vi "제목없음 2.vi"() -> ()   [LabVIEW 2017]
uses:
  <vilib>/DAQmx/read.llb/DAQmx Read (Analog Wfm 1Chan NSamp).vi
  <vilib>/DAQmx/create/channels.llb/DAQmx Create Channel (AI-Voltage-Basic).vi
  <vilib>/DAQmx/configure/timing.llb/DAQmx Timing (Sample Clock).vi
  <vilib>/DAQmx/miscellaneous.llb/DAQmx Fill In Error Info.vi
panel:
  out "RX.CH2":waveform(dbl)(graph)
  in  "sampling rate":dbl=192000.0 caption="Sampling Frequency" format="%0.2f"
  in  "RX Time(sec)":dbl=0.2
  in  "Number of Sample":i32=19200
  in  "수신 채널 설정":tag="Dev3/ai0:1"
  in  "수신 디바이스 이름":tag="Dev3"
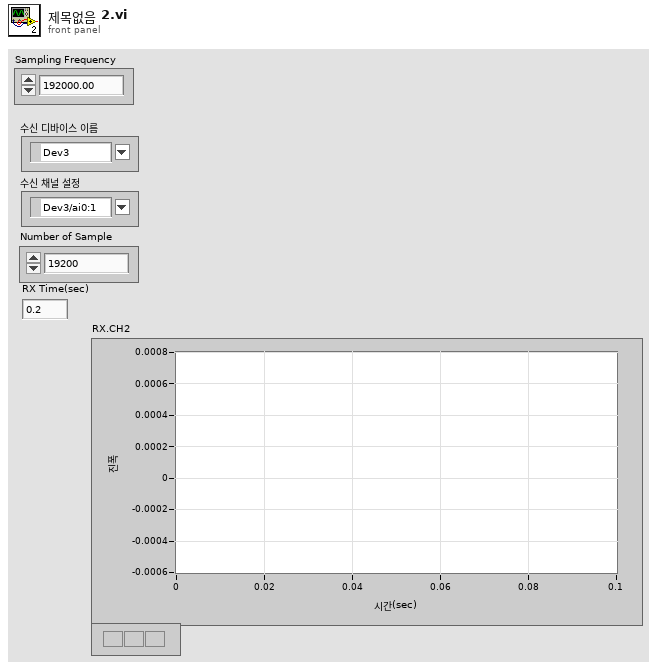
[diagram p1: front panel]
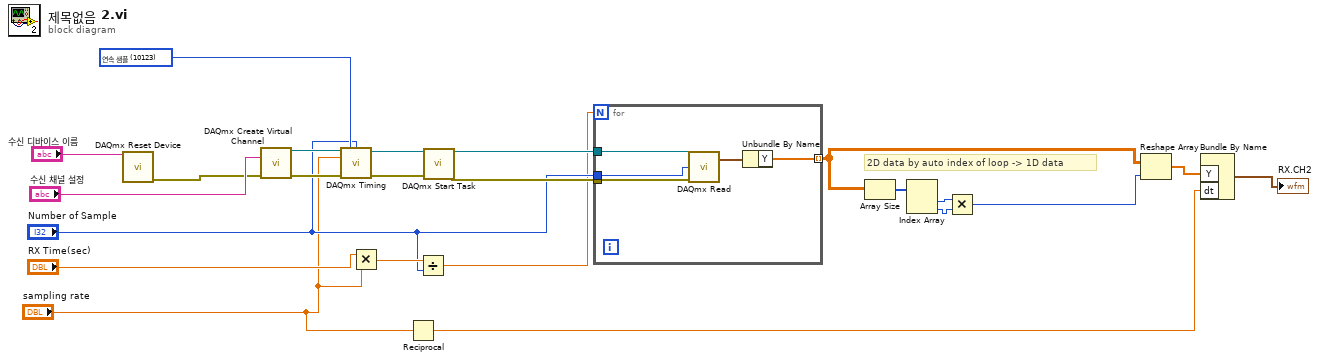
[diagram p0: block diagram]
diagram:
  w14 = 10123 items=["유한 샘플"=10178, "연속 샘플"=10123, "하드웨어 타이밍에 의한 단일 포인트"=12522] ("sample mode")
  # "2D data by auto index of loop -> 1D data"
  n1 = call <vilib>:"DAQmx Reset Device.vi"("device in"="수신 디바이스 이름") -> ("error out"=w20:errorcluster)  [unwired: 1 in, 13 out]
  n2 = call-poly <vilib>:"DAQmx Create Virtual Channel.vi"("physical channels"="수신 채널 설정", "error in"=w20) -> ("task out"=w22:refnum<k21>, "error out"=w19:errorcluster)  [unwired: 7 in, 5 out]
  n3 = call-poly <vilib>:"DAQmx Timing.vi"("task/channels in"=w22, "sample mode"=w14, "samples per channel"="Number of Sample", "rate"="sampling rate", "error in"=w19) -> ("task out"=w17:refnum<k21>, "error out"=w18:errorcluster)  [unwired: 2 in, 7 out]
  n4 = Multiply(x="RX Time(sec)", y="sampling rate") -> (x*y=w12:dbl)
  n5 = Reciprocal(x="sampling rate") -> (1/x=w3:dbl)
  n6 = Divide(x=w12, y="Number of Sample") -> (x/y=w10:dbl)
  n7 = call <vilib>:"DAQmx Start Task.vi"("task/channels in"=w17, "error in"=w18) -> ("task out"=w16:refnum<k21>, "error out"=w15:errorcluster)  [unwired: 12 in]
  n8 = for {
    N: w10 -> [_]
    tunnel: w16 -> [w28]
    tunnel: w15 -> [w27]
    tunnel: "Number of Sample" -> [w26]
    tunnel: [w24] -> w6 mode=indexing
    n9 = call-poly <vilib>:"DAQmx Read.vi"("task/channels in"=w28, "number of samples per channel"=w26, "error in"=w27) -> ("data"=w25:waveform(dbl))  [unwired: 12 out]
    n10 = Unbundle By Name(w25) -> ("Y"=w24:dbl[])
  }
  n11 = Array Size(array=w6) -> (size(s)=w7:i32[])
  n12 = Index Array(array=w7) -> (element #1=w8:i32, element #2=w1:i32)  [unwired: 2 in]
  n13 = Multiply(x=w8, y=w1) -> (x*y=w9:i32)
  n14 = Reshape Array(w6, w9) -> (w5:dbl[])
  n15 = Bundle By Name("Y"=w5, "dt"=w3) -> (→"RX.CH2":waveform(dbl))  [unwired: 1 in]
